vi "GD_Robot_Carrier_num.vi"(8 "error in (no error)":errorcluster, 9 "carrier_num":i32, 10 "glue_data_id":string, 11 "DBlink":string="Driver={ODBC Driver 17 for SQL Server};Server=localhost\\SQLEXPRESS;Database=ZDX201;UID=labview;PWD=Dsa@54137926") -> (0 "error out":errorcluster, 2 "carrier_result":i32)   [LabVIEW 2019]
uses:
  <vilib>/addons/database/Connection.llb/DB Tools Open Connec (String).vi
  <vilib>/addons/database/Connection.llb/Conn Execute.vi
  <vilib>/addons/database/Recordset.llb/Rec Fetch Recordset Data (R).vi
  <vilib>/addons/database/Recordset.llb/Rec Destroy - Connection.vi
  <vilib>/addons/database/_DB Variant To Data/Database Variant To Data.xnode
  <vilib>/addons/database/NI_Database_API.lvlib
panel:
  out "Original num":i32
  out "Command 1":string="SELECT TOP (1) [id]      \n FROM [ZDX201].[dbo].[glue_data]\n where glue_workspace_id=7 and evaluation_2 is not null\norder by id desc "
  out "Command 2":string="WHERE [id]=16"
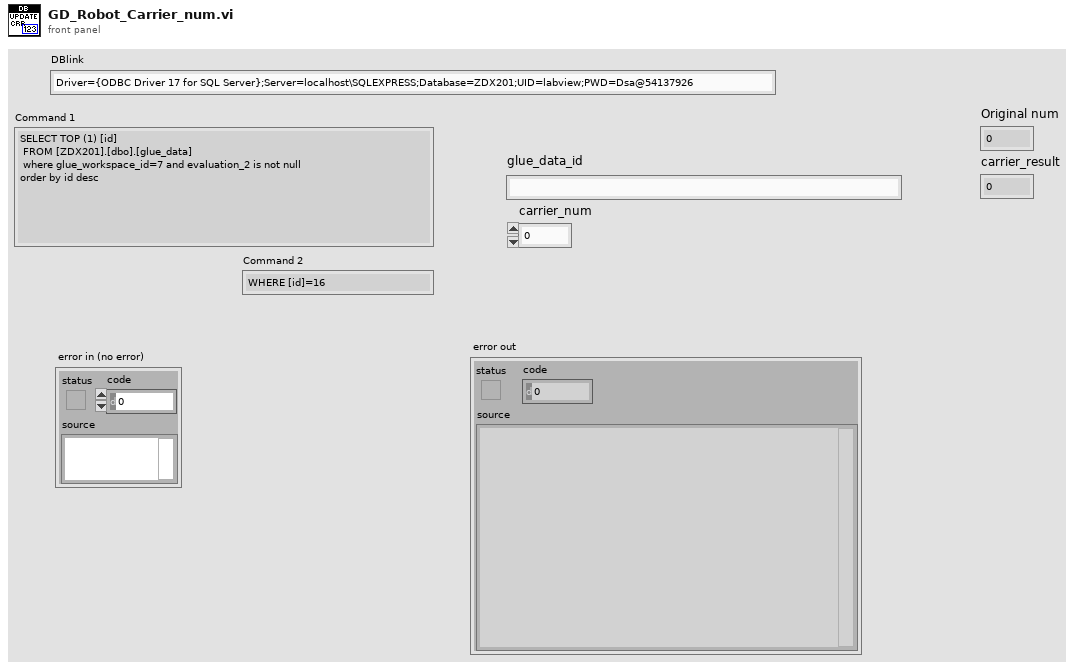
[diagram p1: front panel]
types:
  T1 = cluster{"carrier_num":i32, "update_time":timestamp}
  T2 = typedef "NI_Database_API.lvlib/Conn ObjectReference.ctl" = refnum<k1>
  T3 = typedef "NI_Database_API.lvlib/Rec ObjectReference.ctl" = refnum<k1>
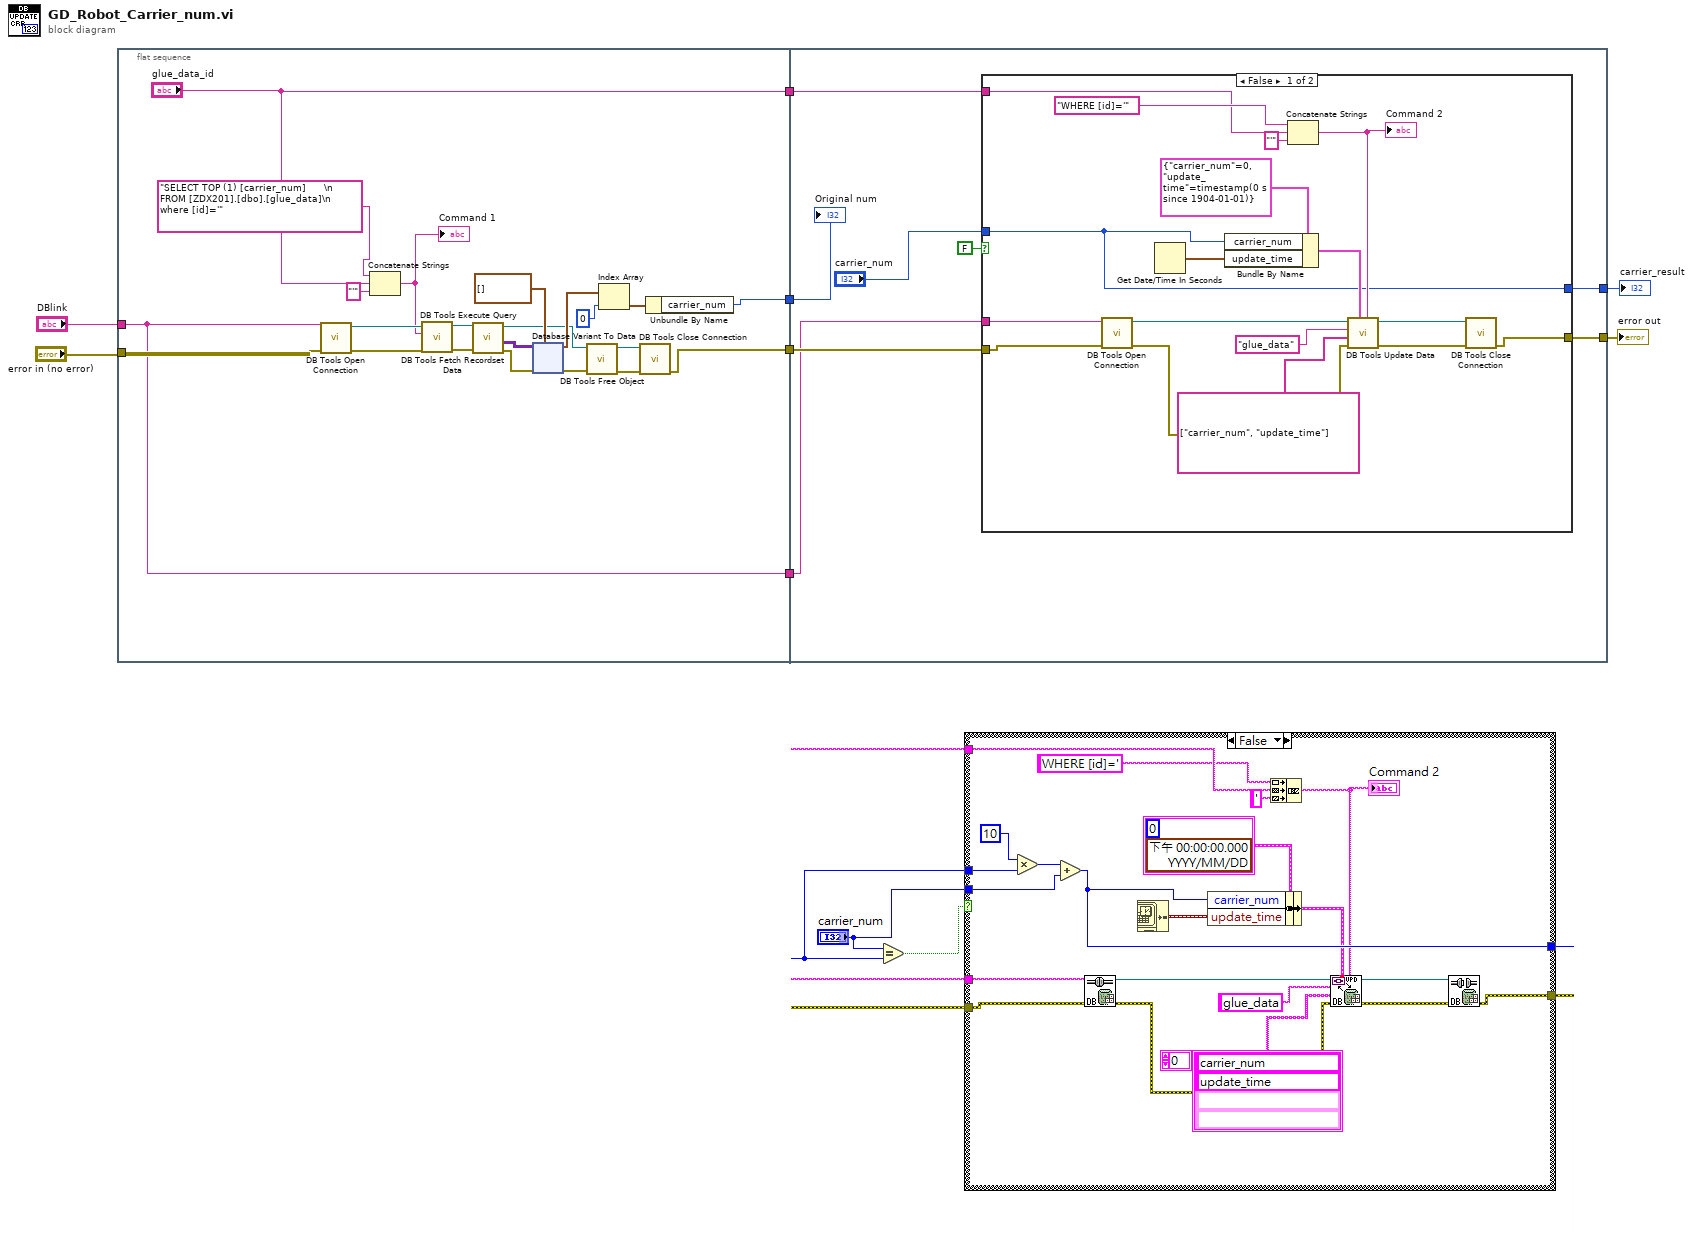
[diagram p0: block diagram]
diagram:
  n1 = flat-sequence {
    tunnel: "DBlink" -> [w16]
    tunnel: "error in (no error)" -> [w30]
    tunnel: [w17] -> w6
    tunnel: [w16] -> w5
    tunnel: [w10] -> w4
    tunnel: ["glue_data_id"] -> w3
    tunnel: w6 -> [w79]
    tunnel: w5 -> [w75]
    tunnel: w4 -> [w72]
    tunnel: w3 -> [w77]
    tunnel: [w76] -> w2
    tunnel: [w74] -> w1
    frame #0 {
      n2 = call-poly <vilib>:"DB Tools Open Connection.vi"("error in (no error)"=w30, "connection information"=w16) -> ("error out"=w29:errorcluster, "connection reference"=w28:T2)  [unwired: 6 in]
      n3 = Concatenate Strings("SELECT TOP (1) [carrier_num]      \n FROM [ZDX201].[dbo].[glue_data]\n where [id]='" ("SQL query"), "glue_data_id", "'" ("string")) -> (w13:string)
      "Command 1" <- w13
      n4 = call-poly <vilib>:"DB Tools Execute Query.vi"("error in (no error)"=w29, "SQL query"=w13, "connection reference"=w28) -> ("error out"=w27:errorcluster, "recordset reference"=w26:T3)  [unwired: 5 in]
      n5 = call-poly <vilib>:"DB Tools Fetch Recordset Data.vi"("error in (no error)"=w27, "recordset reference"=w26) -> ("error out"=w25:errorcluster, "recordset data"=w15:variant[][], "recordset reference out"=w18:T3)  [unwired: 3 in]
      n6 = xnode "Database Variant To Data"("database variant"=w15, "error in (no error)"=w25, "type"=cluster{"carrier_num":i32}[] [] ("initialized array")) -> ("data"=w23:cluster{"carrier_num":i32}[], "error out"=w19:errorcluster)
      n7 = call-poly <vilib>:"DB Tools Free Object.vi"("error in (no error)"=w19, "recordset reference"=w18) -> ("error out"=w20:errorcluster, "connection reference"=w21:T2)  [unwired: 8 in]
      n8 = Index Array(array=w23, index=0) -> (element=w11:cluster{"carrier_num":i32})
      n9 = call <vilib>:"DB Tools Close Connection.vi"("error in (no error)"=w20, "connection reference"=w21) -> ("error out"=w17:errorcluster)  [unwired: 5 in]
      n10 = Unbundle By Name(w11) -> ("carrier_num"=w10:i32)
    }
    frame #1 {
      n11 = case shown="False" FALSE {
        tunnel: w79 -> [w83 w98]
        tunnel: "carrier_num" -> [w80 w97]
        tunnel: w77 -> [w84 _]
        tunnel: [w82 w98] -> w76
        tunnel: w75 -> [w81 _]
        tunnel: [w80 w97] -> w74
        frame False {
          n12 = call-poly <vilib>:"DB Tools Open Connection.vi"("error in (no error)"=w83, "connection information"=w81) -> ("error out"=w91:errorcluster, "connection reference"=w95:T2)  [unwired: 6 in]
          n13 = Get Date/Time In Seconds() -> (seconds since 1Jan1904=w96:timestamp)
          n14 = Bundle By Name(cluster=T1 {"carrier_num"=0, "update_time"=timestamp(0 s since 1904-01-01)}, "carrier_num"=w80, "update_time"=w96) -> (w94:T1)
          n15 = Concatenate Strings("WHERE [id]='", w84, "'" ("string")) -> (w93:string)
          "Command 2" <- w93
          n16 = call <vilib>:"DB Tools Update Data.vi"("condition"=w93, "data"=w94, "error in (no error)"=w91, "columns"=string[] ["carrier_num", "update_time"], "table"="glue_data", "connection reference"=w95) -> ("error out"=w90:errorcluster, "connection reference out"=w92:T2)  [unwired: 4 in]
          n17 = call <vilib>:"DB Tools Close Connection.vi"("error in (no error)"=w90, "connection reference"=w92) -> ("error out"=w82:errorcluster)  [unwired: 5 in]
        }
        frame True {
          # "底座號碼一樣沒事"
        }
      }
      "Original num" <- w72
    }
  }
  "error out" <- w2
  "carrier_result" <- w1
